vi "Dynamic Load  Line Detector.vi"(8 "Error In":errorcluster) -> (0 "Error Out":errorcluster, 3 "Module":refnum<class "Template Module.lvclass">)   [LabVIEW 2016]
uses:
  Template Module/Template Module.lvclass
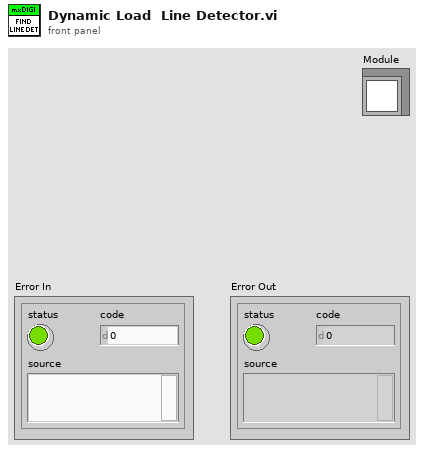
[diagram p1: front panel]
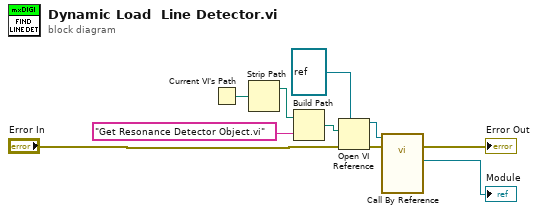
[diagram p0: block diagram]
diagram:
  n1 = Current VI's Path() -> (path=w6:path)
  n2 = Strip Path(path=w6) -> (stripped path=w1:path)  [unwired: 1 out]
  n3 = Build Path(base path=w1, name or relative path="Get Resonance Detector Object.vi") -> (appended path=w2:path)
  n4 = Open VI Reference(type specifier VI Refnum (for type only)=refnum<vi> refnum, vi path=w2, error in (no error)="Error In") -> (vi reference=w4:refnum<vi>, error out=w3:errorcluster)  [unwired: 3 in]
  n5 = call-by-ref "?"(reference=w4, error in=w3) -> (error out=→"Error Out":errorcluster, "Module"=→"Module":refnum<class "Template Module.lvclass">)  [unwired: 11 in, 1 out]
